vi "Compress LIDAR Data.vi"(8 "Compression Factor":i32, 10 "Direction":dbl[](array[numeric]), 11 "Magnitude":dbl[](array[numeric])) -> (2 "Compressed Direction":dbl[](array[numeric]), 3 "Compressed Magnitude":dbl[](array[numeric]))   [LabVIEW 2012]
panel:
  # "NOTE - input directions are assumed to be sorted!"
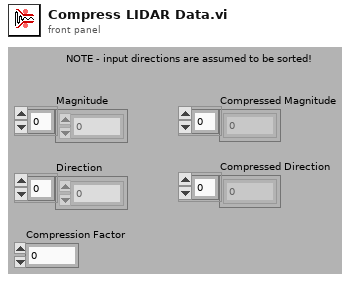
[diagram p1: front panel]
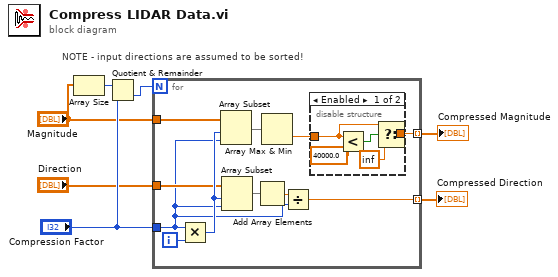
[diagram p0: block diagram]
diagram:
  # "NOTE - input directions are assumed to be sorted!"
  n1 = Array Size(array="Magnitude") -> (size(s)=w1:i32)
  n2 = Quotient & Remainder(x=w1, y="Compression Factor") -> (floor(x/y)=w2:i32)  [unwired: 1 out]
  n3 = for {
    N: w2 -> [_]
    tunnel: "Magnitude" -> [w18]
    tunnel: "Direction" -> [w15]
    tunnel: "Compression Factor" -> [w12]
    tunnel: [w8] -> w7 mode=indexing
    tunnel: [w10] -> w6 mode=indexing
    i -> [w17]
    n4 = Multiply(x=w12, y=w17) -> (x*y=w16:i32)
    n5 = Array Subset(array=w18, index=w16, length=w12) -> (w11:dbl[])
    n6 = Array Subset(array=w15, index=w16, length=w12) -> (w14:dbl[])
    n7 = Add Array Elements(numeric array=w14) -> (sum=w13:dbl)
    n8 = Array Max & Min(array=w11) -> (min value=w9:dbl)  [unwired: 3 out]
    n9 = Divide(x=w13, y=w12) -> (x/y=w10:dbl)
    n10 = disable-structure shown="Enabled" {
      disable-tunnel: w9 -> [w22 w24]
      disable-tunnel: [w20 w24] -> w8
      frame Enabled {
        n11 = Less?(x=w22, y=40000.0) -> (x < y?=w19:bool)
        n12 = Select(t=w22, s=w19, f=inf) -> (s? t:f=w20:dbl)
      }
      frame Disabled {
      }
    }
  }
  "Compressed Magnitude" <- w7
  "Compressed Direction" <- w6
